vi "HitrapGUI.showMCPValues.vi"(0 "Cluster Refnum":refnum<vi>, 2 "show":bool, 5 "error in (no error)":errorcluster) -> (14 "Cluster Refnum Out":refnum<vi>, 19 "error out":errorcluster)   [LabVIEW 2014, in "HitrapGUI.lvlib"]
uses:
  HitrapGUI.lvlib
panel:
  in  "numericType":dbl
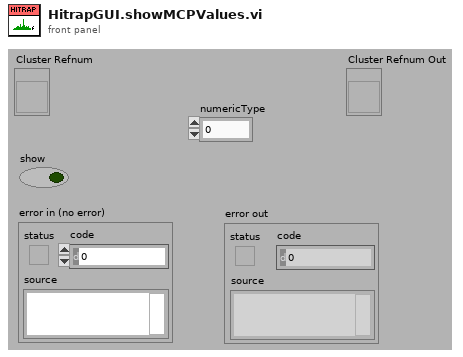
[diagram p1: front panel]
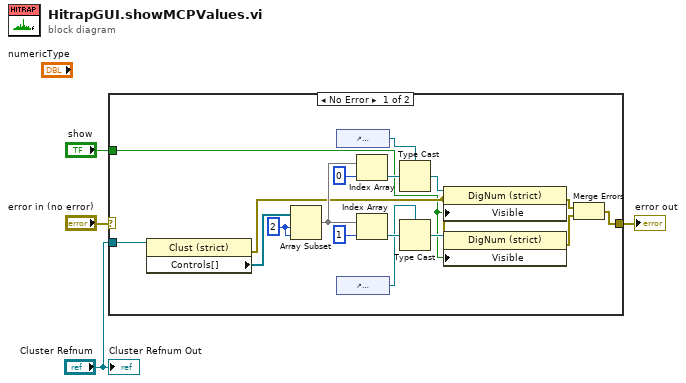
[diagram p0: block diagram]
diagram:
  n1 = case shown="No Error" "error in (no error)" {
    selector: "error in (no error)" -> [_ w22]
    tunnel: "show" -> [w9 _]
    tunnel: "Cluster Refnum" -> [w20 _]
    tunnel: [w5 w22] -> w2
    frame No Error {
      w19 = 2 ("index")
      n2 = property class="Clust (strict)"(reference=w20) -> (error out=w10:errorcluster, "Controls[]"=w21:refnum<vi>[])  [unwired: 1 in, 1 out]
      n3 = Array Subset(array=w21, index=w19, length=w19) -> (w13:refnum<vi>[])
      n4 = control-ref of="numericType"() -> (w17:refnum<vi>)
      n5 = control-ref of="numericType"() -> (w8:refnum<vi>)
      n6 = Index Array(array=w13, index=0) -> (element=w15:refnum<vi>)
      n7 = Index Array(array=w13, index=1) -> (element=w11:refnum<vi>)
      n8 = Type Cast(type=w17, x=w15) -> (*(type *) &x=w18:refnum<vi>)
      n9 = Type Cast(type=w8, x=w11) -> (*(type *) &x=w12:refnum<vi>)
      n10 = property class="DigNum (strict)"(reference=w18, error in=w10, "Visible"=w9) -> (error out=w6:errorcluster)  [unwired: 1 out]
      n11 = property class="DigNum (strict)"(reference=w12, error in=w10, "Visible"=w9) -> (error out=w7:errorcluster)  [unwired: 1 out]
      n12 = Merge Errors(w6, w7) -> (w5:errorcluster)
    }
    frame Error {
    }
  }
  "error out" <- w2
  "Cluster Refnum Out" <- "Cluster Refnum"
